vi "write_params.vi"(8 "error in (no error)":errorcluster, 10 "params":T1={"alpha"=1.0, "fit_intercept"=TRUE, "normalize"=FALSE, "copy_X"=TRUE, "max_iter"=1000.0, "tol"=0.0001, "warm_start"=FALSE, "random_state"=0.0, "selection"="cyclic"}, 11 "MultiTaskLasso in":refnum<class "MultiTaskLasso.lvclass">) -> (0 "error out":errorcluster, 3 "MultiTaskLasso out":refnum<class "MultiTaskLasso.lvclass">)   [LabVIEW 2020, in "MultiTaskLasso.lvclass"]
uses:
  MultiTaskLasso.lvclass
  Controls/multi_task_lasso_params.ctl
  MultiTaskLasso.lvclass/MultiTaskLasso.ctl
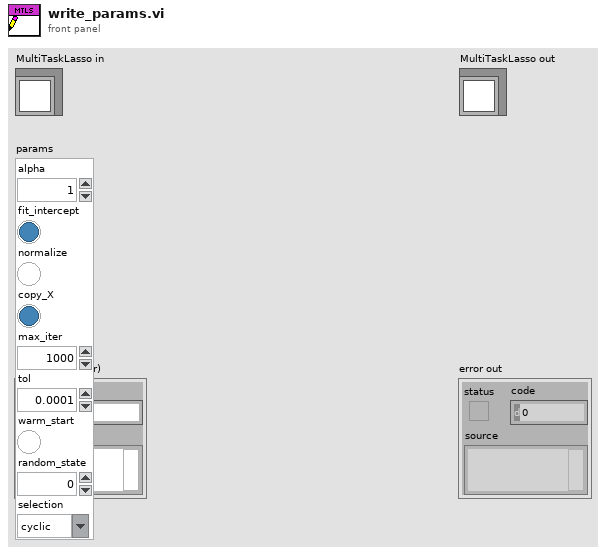
[diagram p1: front panel]
types:
  T1 = typedef "multi_task_lasso_params.ctl" = cluster{"alpha":dbl, "fit_intercept":bool, "normalize":bool, "copy_X":bool, "max_iter":dbl, "tol":dbl, "warm_start":bool, "random_state":dbl, "selection":string}
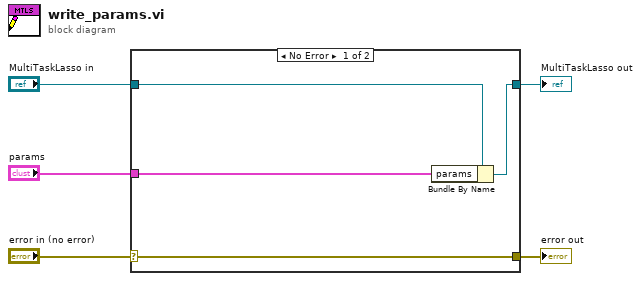
[diagram p0: block diagram]
diagram:
  n1 = case shown="No Error" "error in (no error)" {
    selector: "error in (no error)" -> [w9 w10]
    tunnel: [w9 w10] -> w4
    tunnel: [w7 w11] -> w2
    tunnel: "MultiTaskLasso in" -> [w8 w11]
    tunnel: "params" -> [w6 _]
    frame No Error {
      n2 = Bundle By Name(cluster=w8, "params"=w6) -> (w7:refnum<class "MultiTaskLasso.lvclass">)
    }
    frame Error {
    }
  }
  "error out" <- w4
  "MultiTaskLasso out" <- w2
